vi "anna_auto_spotfindsettings.vi"(7 "Enum":T2(ring), 9 "already x spots found":i16, 11 "notes 2":refnum<vi>) -> (0 "settings":string, 2 "spotfinding settings":T1={"show all"=FALSE, "threshold/morph"=FALSE, "particle filter"=FALSE, "spot marks"=FALSE, "close filter"=FALSE, "connectivity 4/8"=FALSE, "range"={"Lower value"=30.0, "Upper value"=30.0}, "PSF-size"=0, "Parameters"=[]} {"range"."Upper value" format="%.2f"; "range"."Lower value" format="%.2f"; "Parameters"."Upper Value" format="%.2f"; "Parameters"."Lower Value" format="%.2f"}, 4 "coordinates":i32[][](array[numeric]))   [LabVIEW 2009]
uses:
  spotfindersettings.ctl
panel:
  out "Number of Particles":i32
  in  "UPDATE":bool
  in  "notes":string
  # "Selection Values"
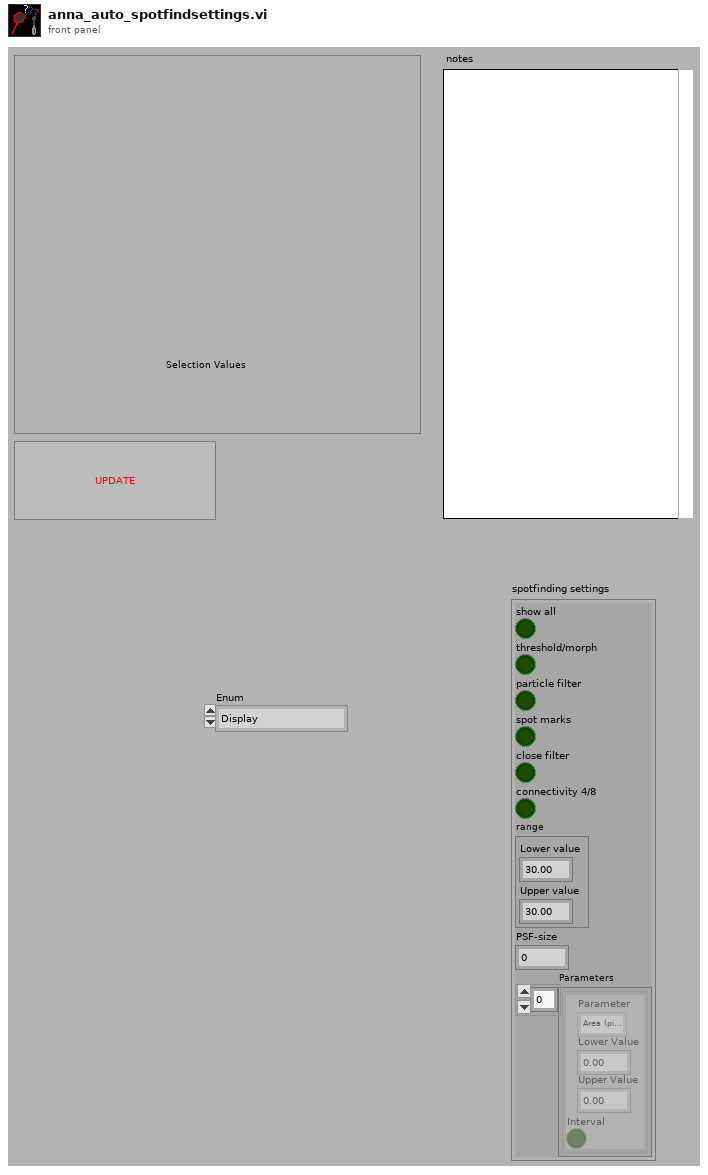
[diagram p1: front panel]
types:
  T1 = typedef "spotfindersettings.ctl" = cluster{"show all":bool, "threshold/morph":bool, "particle filter":bool, "spot marks":bool, "close filter":bool, "connectivity 4/8":bool, "range":cluster{"Lower value":sgl, "Upper value":sgl}, "PSF-size":i32, "Parameters":cluster{"Parameter":enum32{"Area (pixels)", "Area (calibrated)", "Number of holes", "Holes area (pixels)", "Total area (pixels)", "Scanned area (pixels)", "Ratio Area/Scanned area (%)", "Ratio Area/Total area (%)", "Center of mass (X)", "Center of mass (Y)", "Left column (X)", "Upper row (Y)", "Right column (X)", "Lower row (Y)", "Width (pixels)", "Height (pixels)", "Longest segment length", "Longest segment left column (X)", "Longest segment top row  (Y)", "Perimeter", "Holes perimeter", "SumX", "SumY", "SumXX", "SumYY", "SumXY", "Corrected projection X", "Corrected projection Y", "Moment of inertia Ixx", "Moment of inertia Iyy", "Moment of inertia Ixy", "Mean chord X", "Mean chord Y", "Max intercept", "Mean intercept perpendicular", "Particle orientation", "Equivalent ellipse minor axis", "Ellipse major axis", "Ellipse minor axis", "Ratio of equivalent ellipse axis", "Rectangle big side", "Rectangle small side", "Ratio of equivalent rectangle sides", "Elongation factor", "Compactness factor", "Heywood circularity factor", "Type factor", "Hydraulic radius", "Waddel disk diameter", "Diagonal"}, "Lower Value":sgl, "Upper Value":sgl, "Interval":bool}[]}
  T2 = enum16{"Display", "change", "get", "save", "create text", "load", "Get Refnum"}
  T3 = enum16{"Ini", "Get", "Set", "Refresh", "dump", "move", "name"}
  T4 = typedef "IMAQ Image.ctl" = refnum<image>
  T5 = cluster{"Parameter":enum32{"Area (pixels)", "Area (calibrated)", "Number of holes", "Holes area (pixels)", "Total area (pixels)", "Scanned area (pixels)", "Ratio Area/Scanned area (%)", "Ratio Area/Total area (%)", "Center of mass (X)", "Center of mass (Y)", "Left column (X)", "Upper row (Y)", "Right column (X)", "Lower row (Y)", "Width (pixels)", "Height (pixels)", "Longest segment length", "Longest segment left column (X)", "Longest segment top row  (Y)", "Perimeter", "Holes perimeter", "SumX", "SumY", "SumXX", "SumYY", "SumXY", "Corrected projection X", "Corrected projection Y", "Moment of inertia Ixx", "Moment of inertia Iyy", "Moment of inertia Ixy", "Mean chord X", "Mean chord Y", "Max intercept", "Mean intercept perpendicular", "Particle orientation", "Equivalent ellipse minor axis", "Ellipse major axis", "Ellipse minor axis", "Ratio of equivalent ellipse axis", "Rectangle big side", "Rectangle small side", "Ratio of equivalent rectangle sides", "Elongation factor", "Compactness factor", "Heywood circularity factor", "Type factor", "Hydraulic radius", "Waddel disk diameter", "Diagonal"}, "Lower Value":sgl, "Upper Value":sgl, "Interval":bool}[]
  T6 = enum32{"Area (pixels)", "Area (calibrated)", "Number of holes", "Holes area (pixels)", "Total area (pixels)", "Scanned area (pixels)", "Ratio Area/Scanned area (%)", "Ratio Area/Total area (%)", "Center of mass (X)", "Center of mass (Y)", "Left column (X)", "Upper row (Y)", "Right column (X)", "Lower row (Y)", "Width (pixels)", "Height (pixels)", "Longest segment length", "Longest segment left column (X)", "Longest segment top row  (Y)", "Perimeter", "Holes perimeter", "SumX", "SumY", "SumXX", "SumYY", "SumXY", "Corrected projection X", "Corrected projection Y", "Moment of inertia Ixx", "Moment of inertia Iyy", "Moment of inertia Ixy", "Mean chord X", "Mean chord Y", "Max intercept", "Mean intercept perpendicular", "Particle orientation", "Equivalent ellipse minor axis", "Ellipse major axis", "Ellipse minor axis", "Ratio of equivalent ellipse axis", "Rectangle big side", "Rectangle small side", "Ratio of equivalent rectangle sides", "Elongation factor", "Compactness factor", "Heywood circularity factor", "Type factor", "Hydraulic radius", "Waddel disk diameter", "Diagonal"}
  T7 = cluster{"show all":bool, "threshold/morph":bool, "particle filter":bool, "spot marks":bool, "close filter":bool, "connectivity 4/8":bool, "range":cluster{"Lower value":sgl, "Upper value":sgl}, "PSF-size":i32, "Parameters":cluster{"Parameter":enum32{"Area (pixels)", "Area (calibrated)", "Number of holes", "Holes area (pixels)", "Total area (pixels)", "Scanned area (pixels)", "Ratio Area/Scanned area (%)", "Ratio Area/Total area (%)", "Center of mass (X)", "Center of mass (Y)", "Left column (X)", "Upper row (Y)", "Right column (X)", "Lower row (Y)", "Width (pixels)", "Height (pixels)", "Longest segment length", "Longest segment left column (X)", "Longest segment top row  (Y)", "Perimeter", "Holes perimeter", "SumX", "SumY", "SumXX", "SumYY", "SumXY", "Corrected projection X", "Corrected projection Y", "Moment of inertia Ixx", "Moment of inertia Iyy", "Moment of inertia Ixy", "Mean chord X", "Mean chord Y", "Max intercept", "Mean intercept perpendicular", "Particle orientation", "Equivalent ellipse minor axis", "Ellipse major axis", "Ellipse minor axis", "Ratio of equivalent ellipse axis", "Rectangle big side", "Rectangle small side", "Ratio of equivalent rectangle sides", "Elongation factor", "Compactness factor", "Heywood circularity factor", "Type factor", "Hydraulic radius", "Waddel disk diameter", "Diagonal"}, "Lower Value":sgl, "Upper Value":sgl, "Interval":bool}[]}
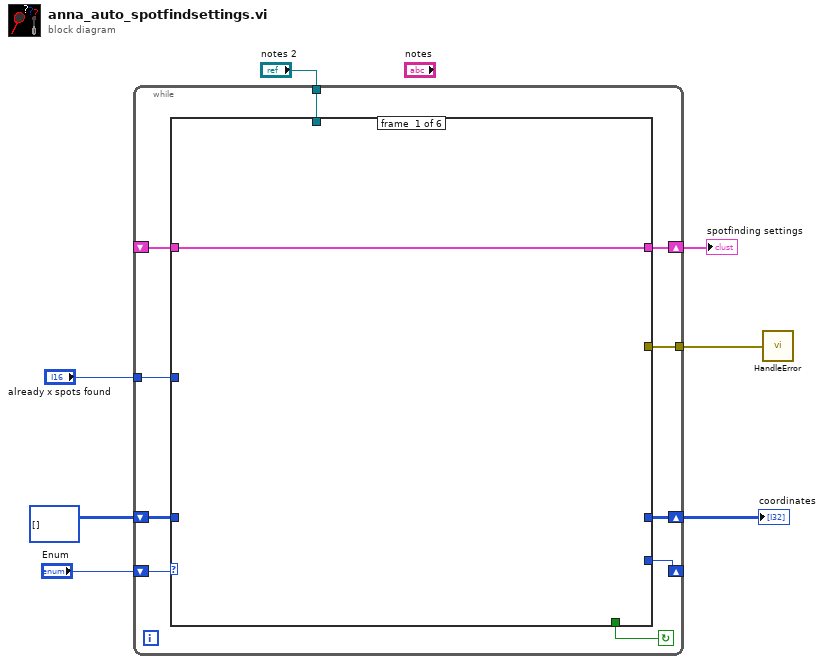
[diagram p0: block diagram]
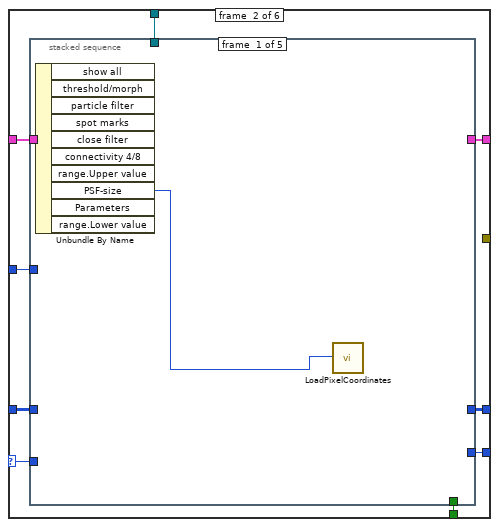
[diagram p2: hidden frame]
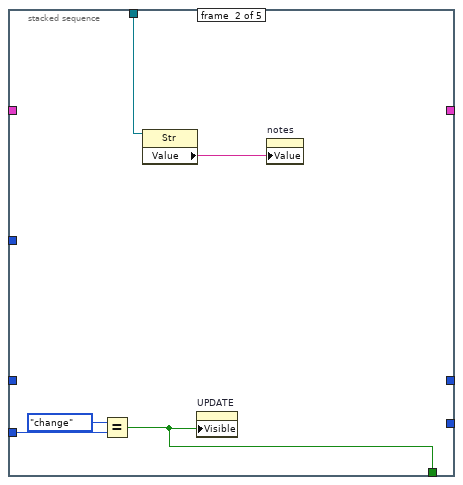
[diagram p3: hidden frame]
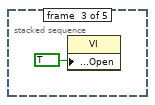
[diagram p4: hidden frame]
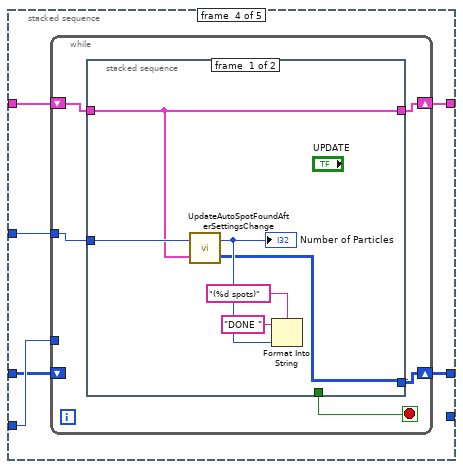
[diagram p5: hidden frame]
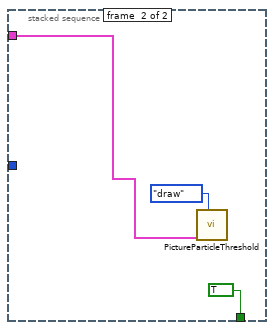
[diagram p6: hidden frame]
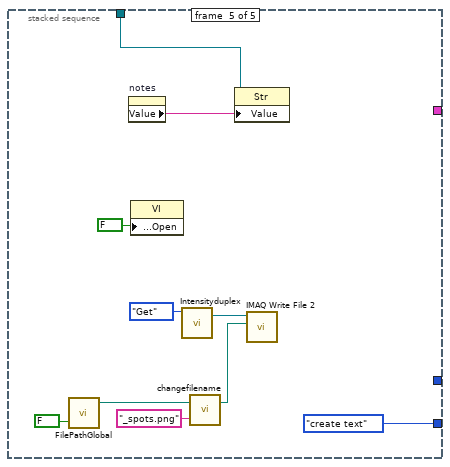
[diagram p7: hidden frame]
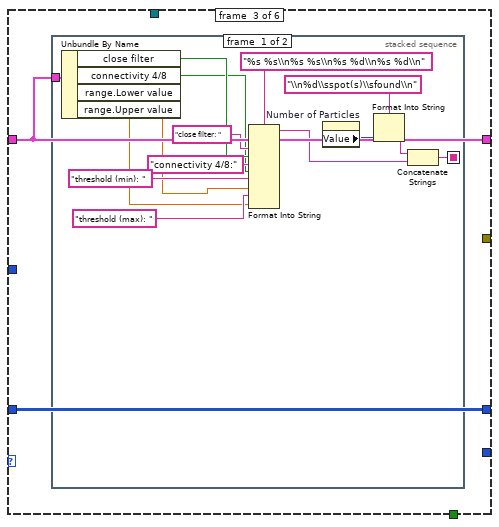
[diagram p8: hidden frame]
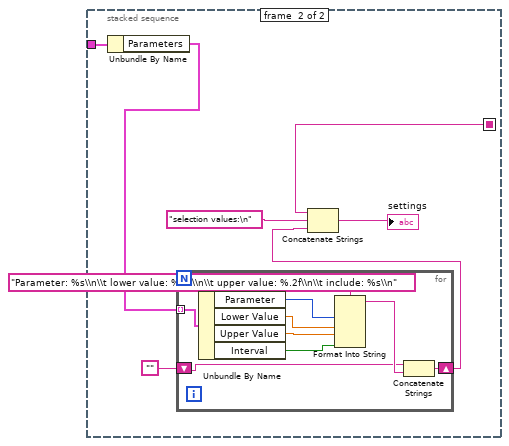
[diagram p9: hidden frame]
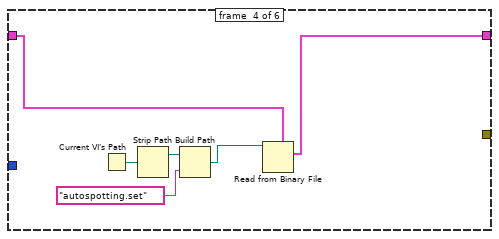
[diagram p10: hidden frame]
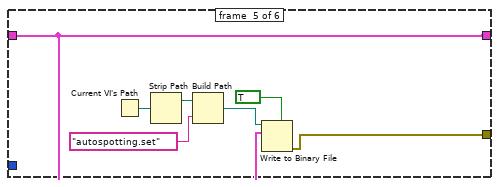
[diagram p11: hidden frame]
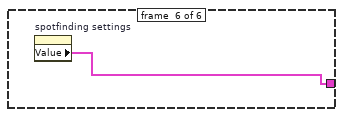
[diagram p12: hidden frame]
diagram:
  n1 = while {
    shift-right: [w8] -> w2
    shift-left: _ -> [w9]
    tunnel: [w17] -> w1
    tunnel: "notes 2" -> [w16]
    tunnel: "already x spots found" -> [w15]
    shift-right: [w12] -> _
    shift-left: "Enum" -> [w13]
    shift-right: [w10] -> w3
    shift-left: i32[][] [] ("coordinates") -> [w11]
    stop <- w14 continue-if-true
    n2 = case shown="\"Display\", \"change\"" w13 {
      selector: w13 -> [_ w21 _ _ _ _]
      tunnel: w9 -> [w18 w27 w66 w99 w105 _]
      tunnel: [_ _ _ _ w107 _] -> w17
      tunnel: w16 -> [_ w26 _ _ _ _]
      tunnel: w15 -> [_ w25 _ _ _ _]
      tunnel: [_ w24 _ _ _ _] -> w14
      tunnel: [_ w23 _ _ _ _] -> w12
      tunnel: [_ w22 w67 _ _ _] -> w10
      tunnel: w11 -> [_ w20 w67 _ _ _]
      tunnel: [w18 w19 w66 w100 w105 w112] -> w8
      frame #0 {
      }
      frame #1 {
        n3 = stacked-sequence {
          tunnel: w27 -> [w29 _ _ w41 _]
          tunnel: [_ _ _ w40 _] -> w19
          tunnel: w26 -> [_ w34 _ _ w63]
          tunnel: w25 -> [_ _ _ w39 _]
          tunnel: [_ w30 _ _ _] -> w24
          tunnel: [_ _ _ _ T2."create text" ("Enum")] -> w23
          tunnel: [_ _ _ w37 _] -> w22
          tunnel: w21 -> [_ w32 _ w38 _]
          tunnel: w20 -> [_ _ _ w36 _]
          frame #0 {
            n4 = Unbundle By Name(w29) -> ("PSF-size"=w28:i32)  [unwired: 9 out]
            n5 = call "LoadPixelCoordinates.vi"("spotsize (radius pixel)"=w28) -> ()
          }
          frame #1 {
            n6 = Equal?(x=T2."change", y=w32) -> (x = y?=w30:bool)
            n7 = property class="Str"(reference=w34) -> ("Value"=w33:string)  [unwired: 1 in, 2 out]
            n8 = property on="UPDATE" class="Bool"("Visible"=w30) -> ()  [unwired: 2 in, 2 out]
            n9 = property on="notes" class="String"("Value"=w33) -> ()  [unwired: 2 in, 2 out]
          }
          frame #2 {
            n10 = property class="VI"("Front Panel Window:Open"=TRUE) -> ()  [unwired: 2 in, 2 out]
          }
          frame #3 {
            n11 = while {
              shift-right: [w43] -> w40
              shift-left: w41 -> [w46]
              tunnel: w39 -> [w45]
              tunnel: w38 -> [_]
              shift-right: [w44] -> w37
              shift-left: w36 -> [_]
              stop <- w42 stop-if-true
              n12 = stacked-sequence {
                tunnel: w46 -> [w47 w55]
                tunnel: w45 -> [w49 _]
                tunnel: [w48 _] -> w44
                tunnel: [w47 _] -> w43
                tunnel: [_ TRUE] -> w42
                frame #0 {
                  n13 = call "UpdateAutoSpotFoundAfterSettingsChange.vi"("spotfinding settings"=w47, "already x spots found"=w49) -> ("coordinates"=w48:i32[][], "Number of Particles"=w50:i32)
                  "Number of Particles" <- w50
                  n14 = Format Into String(format string="(%d spots)", initial string="DONE ", w50) -> ()  [unwired: 1 in, 2 out]
                }
                frame #1 {
                  n15 = call "PictureParticleThreshold.vi"("Enum"=enum16{"new", "input", "draw", "dump"}."draw", "spotfinding settings"=w55) -> ()  [unwired: 6 in, 2 out]
                }
              }
            }
          }
          frame #4 {
            n16 = call "FilePathGlobal.vi"("set?"=FALSE) -> ("Image Path 2"=w58:path)  [unwired: 1 in, 2 out]
            n17 = property on="notes" class="Str"() -> ("Value"=w64:string)  [unwired: 2 in, 2 out]
            n18 = property class="VI"("Front Panel Window:Open"=FALSE) -> ()  [unwired: 2 in, 2 out]
            n19 = call "Intensityduplex.vi"("Enum"=T3."Get") -> ("Image Duplicate (out)"=w60:T4)  [unwired: 4 in, 1 out]
            n20 = call "changefilename.vi"("suffix"="_spots.png", "path in"=w58) -> ("path out"=w56:path)  [unwired: 1 out]
            n21 = property on="Property Node" class="Str"(reference=w63, "Value"=w64) -> ()  [unwired: 1 in, 2 out]
            n22 = call-poly "IMAQ Write File 2"("File Path"=w56, "Image"=w60) -> ()  [unwired: 8 in, 2 out]
          }
        }
      }
      frame #2 {
        n23 = stacked-sequence {
          seq-local: [w74 _] -> [_ w89]
          tunnel: w66 -> [w78 w87]
          frame #0 {
            n24 = Unbundle By Name(w78) -> ("close filter"=w77:bool, "connectivity 4/8"=w76:bool, "range.Lower value"=w75:sgl, "range.Upper value"=w68:sgl)
            n25 = Format Into String(format string="%s %s\\n%s %s\\n%s %d\\n%s %d\\n", "close filter: ", w77, "connectivity 4/8:" ("input 3"), w76, "threshold (min): ", w75, "threshold (max): ", w68) -> (resulting string=w73:string)  [unwired: 2 in, 1 out]
            n26 = property on="Number of Particles" class="Digital (strict)"() -> ("Value"=w72:i32)  [unwired: 2 in, 2 out]
            n27 = Format Into String(format string="\\n%d\\sspot(s)\\sfound\\n", w72) -> (resulting string=w71:string)  [unwired: 2 in, 1 out]
            n28 = Concatenate Strings(w71, w73) -> (w74:string)
          }
          frame #1 {
            n29 = Unbundle By Name(w87) -> ("Parameters"=w83:T5)
            n30 = for {
              shift-right: [w96] -> w86
              shift-left: "" -> [w97]
              tunnel: w83 -> [w94] mode=indexing
              n31 = Unbundle By Name(w94) -> ("Parameter"=w93:T6, "Lower Value"=w92:sgl, "Upper Value"=w91:sgl, "Interval"=w90:bool)
              n32 = Format Into String(format string="Parameter: %s\\n\\t lower value: %.2f\\n\\t upper value: %.2f\\n\\t include: %s\\n", w93, w92, w91, w90) -> (resulting string=w98:string)  [unwired: 2 in, 1 out]
              n33 = Concatenate Strings(w97, w98) -> (w96:string)
            }
            n34 = Concatenate Strings(w89, "selection values:\n", w86) -> (→"settings":string)
          }
        }
      }
      frame #3 {
        n35 = Current VI's Path() -> (path=w104:path)
        n36 = Strip Path(path=w104) -> (stripped path=w103:path)  [unwired: 1 out]
        n37 = Build Path(base path=w103, name or relative path="autospotting.set") -> (appended path=w101:path)
        n38 = Read from Binary File(5:w99, 11:w101) -> (2:w100:T7)  [unwired: 4 in, 3 out]
      }
      frame #4 {
        n39 = Current VI's Path() -> (path=w111:path)
        n40 = Strip Path(path=w111) -> (stripped path=w110:path)  [unwired: 1 out]
        n41 = Build Path(base path=w110, name or relative path="autospotting.set") -> (appended path=w108:path)
        n42 = Write to Binary File(file (use dialog)=w108, data=w105, 5:TRUE ("prepend array or string size? (T)")) -> (error out=w107:errorcluster)  [unwired: 3 in, 2 out]
      }
      frame #5 {
        n43 = property on="spotfinding settings" class="Clust (strict)"() -> ("Value"=w112:T7)  [unwired: 2 in, 2 out]
      }
    }
  }
  "spotfinding settings" <- w2
  "coordinates" <- w3
  n44 = call "HandleError.vi"("error in (no error)"=w1) -> ()
